vi "beam cup control - old.vi"() -> ()   [LabVIEW 2016, in "Top Level.lvlib"]
doc: "This vi is used to control the cups and apertures in the ams beamline."
uses:
  Top Level.lvlib
  sub-VIs/sub-VIs.lvlib
  controls/beamline sections.lvlib
panel:
  in  "Which Beamline":string(combo)="R45"
  out "R45 detector cup":string="OUT"
  out "R45 detector aperture":string="IN"
  out "R45 switch image cup":string="IN"
  out "R45 switch aperture":string="OUT"
  in  "R30 detector ap":bool=TRUE
  out "R30 detector aperture":string="IN"
  out "R30 Detector cup rd":string="OUT"
  out "R30 switch aperture":string="IN"
  in  "R30 Image ap":bool=TRUE
  out "R30 switch image cup":string="OUT"
  out "analyze image cup rd":string="OUT"
  out "tank exit cup  rd":string="OUT"
  out "tank entrance cup  rd":string="OUT"
  out "low energy cup":string="OUT"
  out "injector image aperture":string="IN"
  out "injector cup":string="OUT"
  in  "r45 det cup":bool
  in  "R45  det ap":bool
  in  "r45 switch image cup":bool=TRUE
  in  "R45 #1 ap":bool
  out "Terminal Voltage":dbl=8.333384070396422 format="%#_4g"
  in  "R30 det cup":bool
  in  "Switch magnet cup":bool
  in  "Analyze image cup":bool
  in  "Tank exit cup":bool
  in  "Tank Entrance cup":bool
  in  "Low end waist  cup":bool=TRUE
  in  "Low end waist ap":bool
  in  "INJ Image ap":bool
  in  "Inj Image cup":bool
  out "date/time string":string="3/16/2012  11:07 AM"
  out "Error out":errorcluster
  in  "stop":bool
  # "Faraday cup Controls"
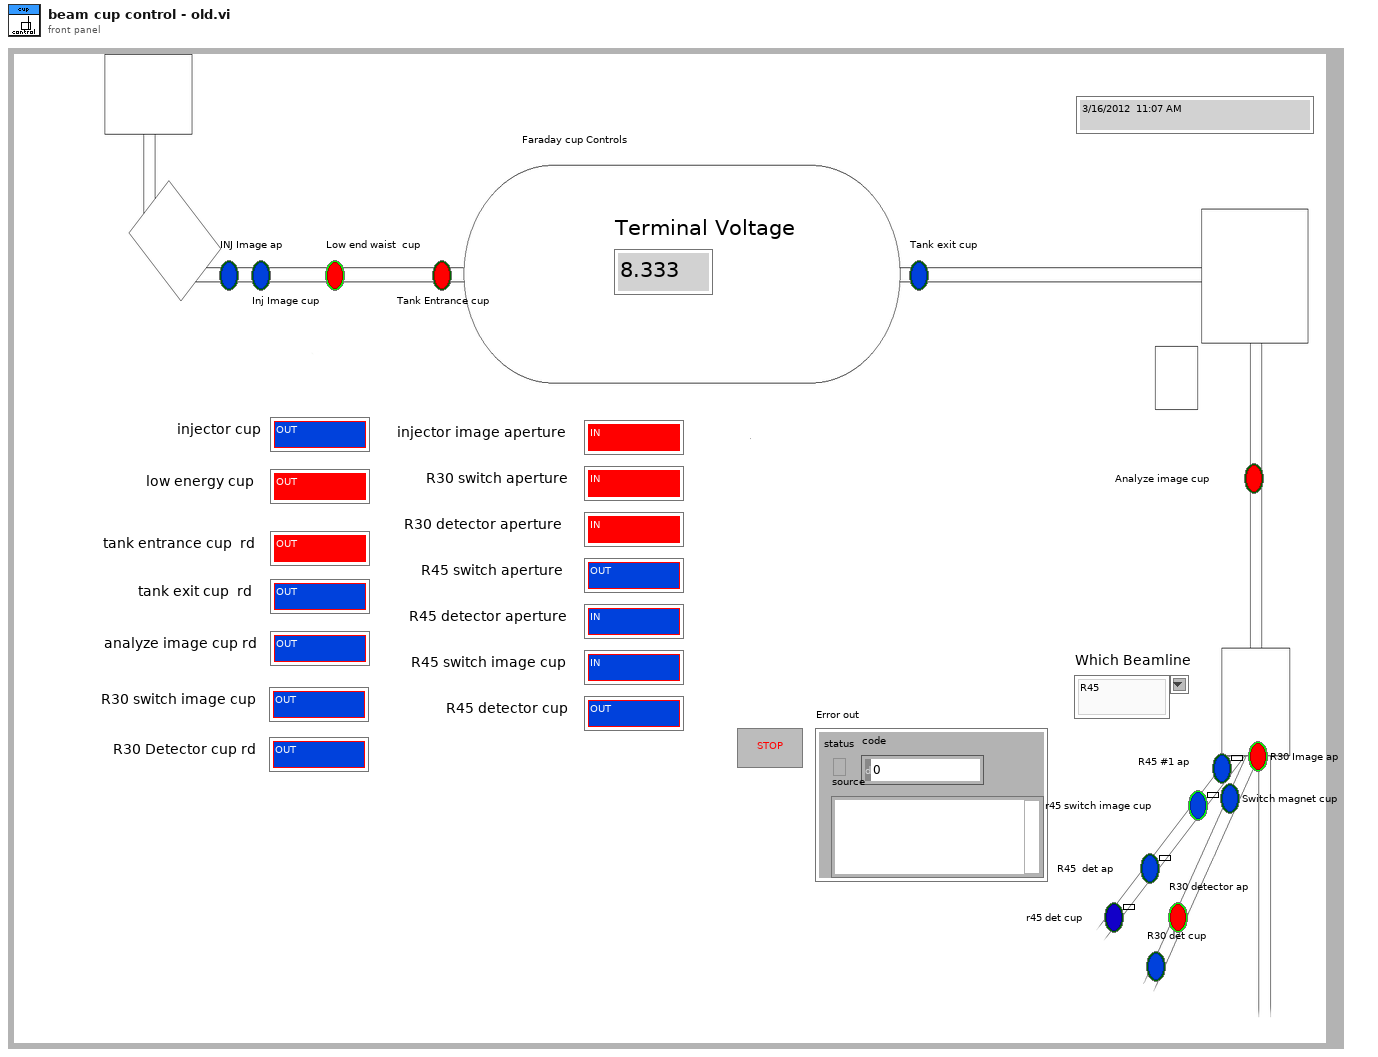
[diagram p1: front panel]
types:
  T1 = typedef "Aperture states.ctl" = enum16{"Aperture status unclear", "Aperture in", "Aperture out"}
  T2 = typedef "Faraday cup states.ctl" = enum16{"FC status unclear", "FC in", "FC out"}
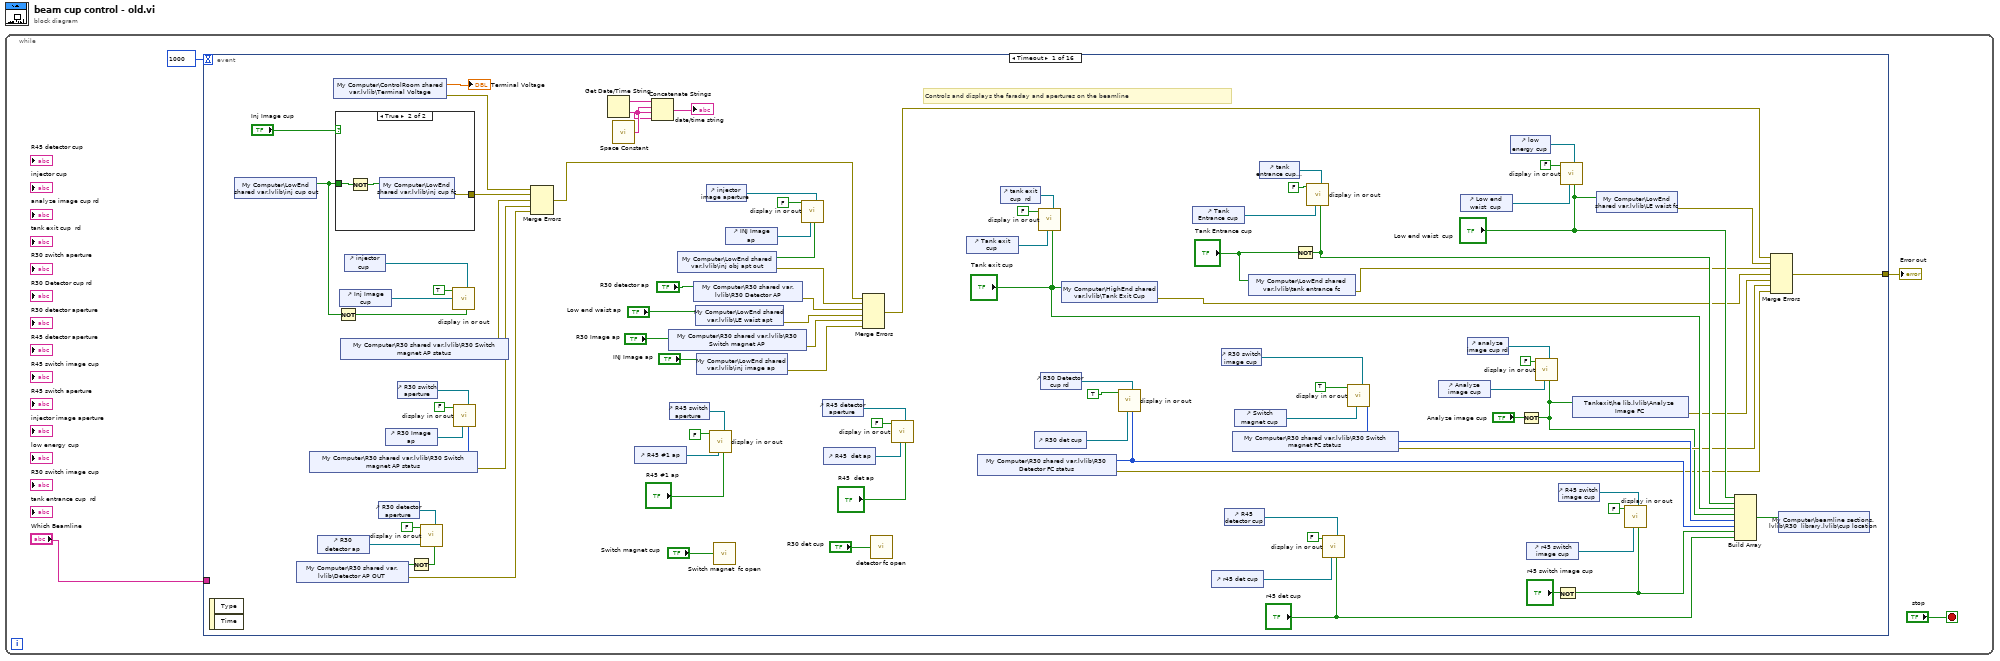
[diagram p0: block diagram]
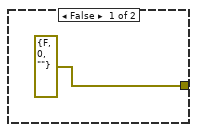
[diagram p2: hidden frame]
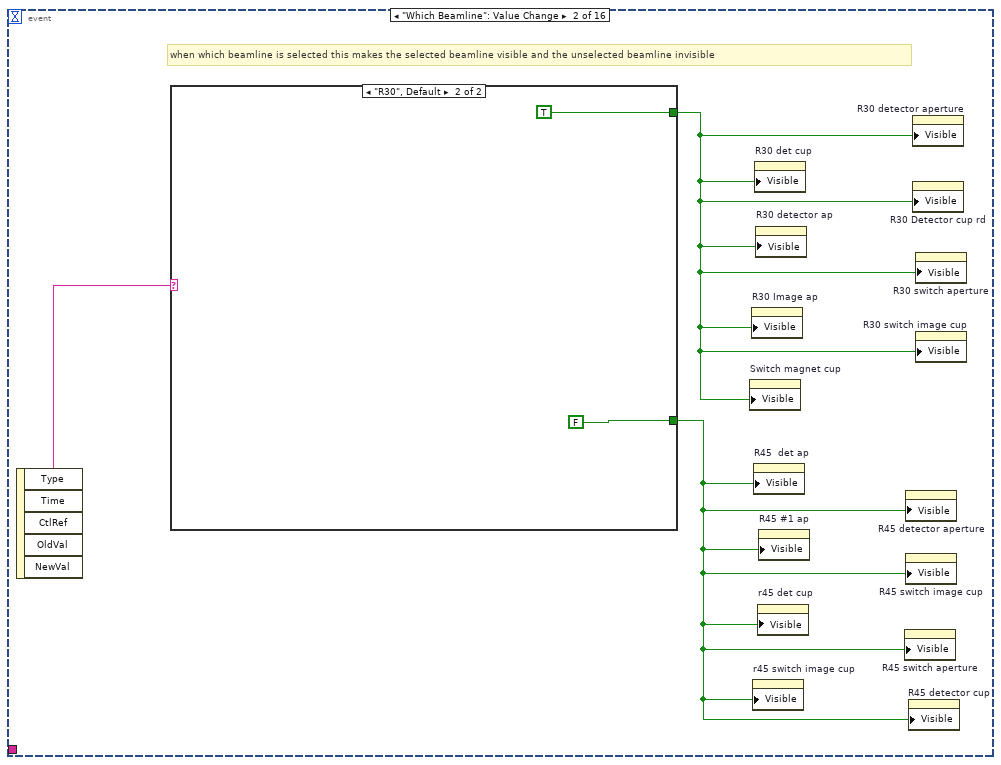
[diagram p3: hidden frame]
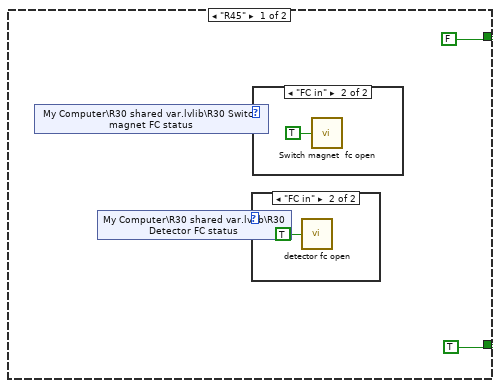
[diagram p4: hidden frame]
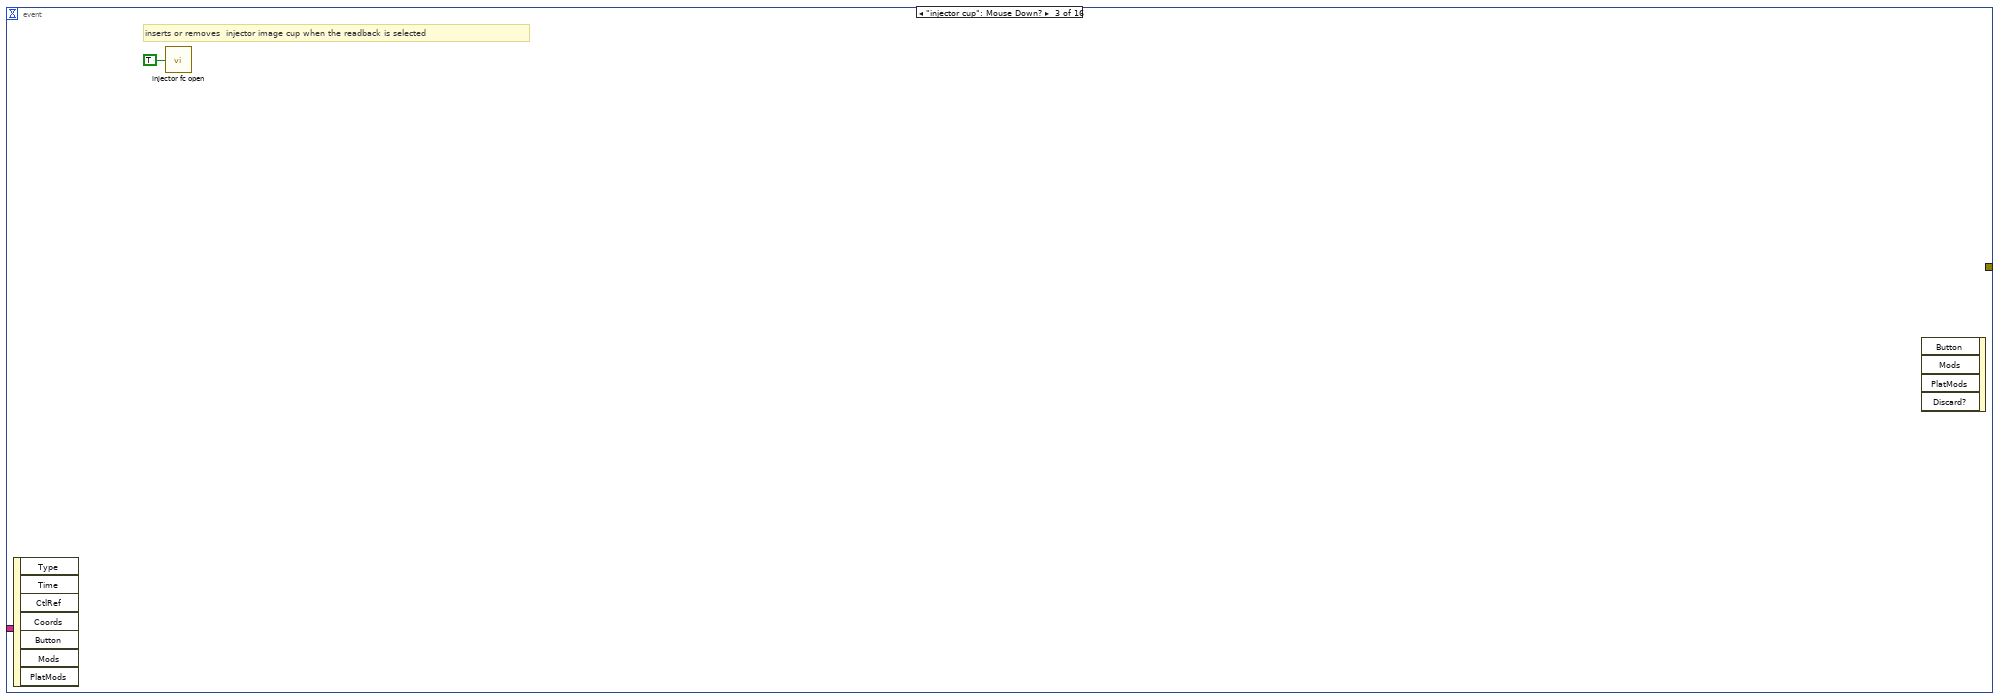
[diagram p7: hidden frame]
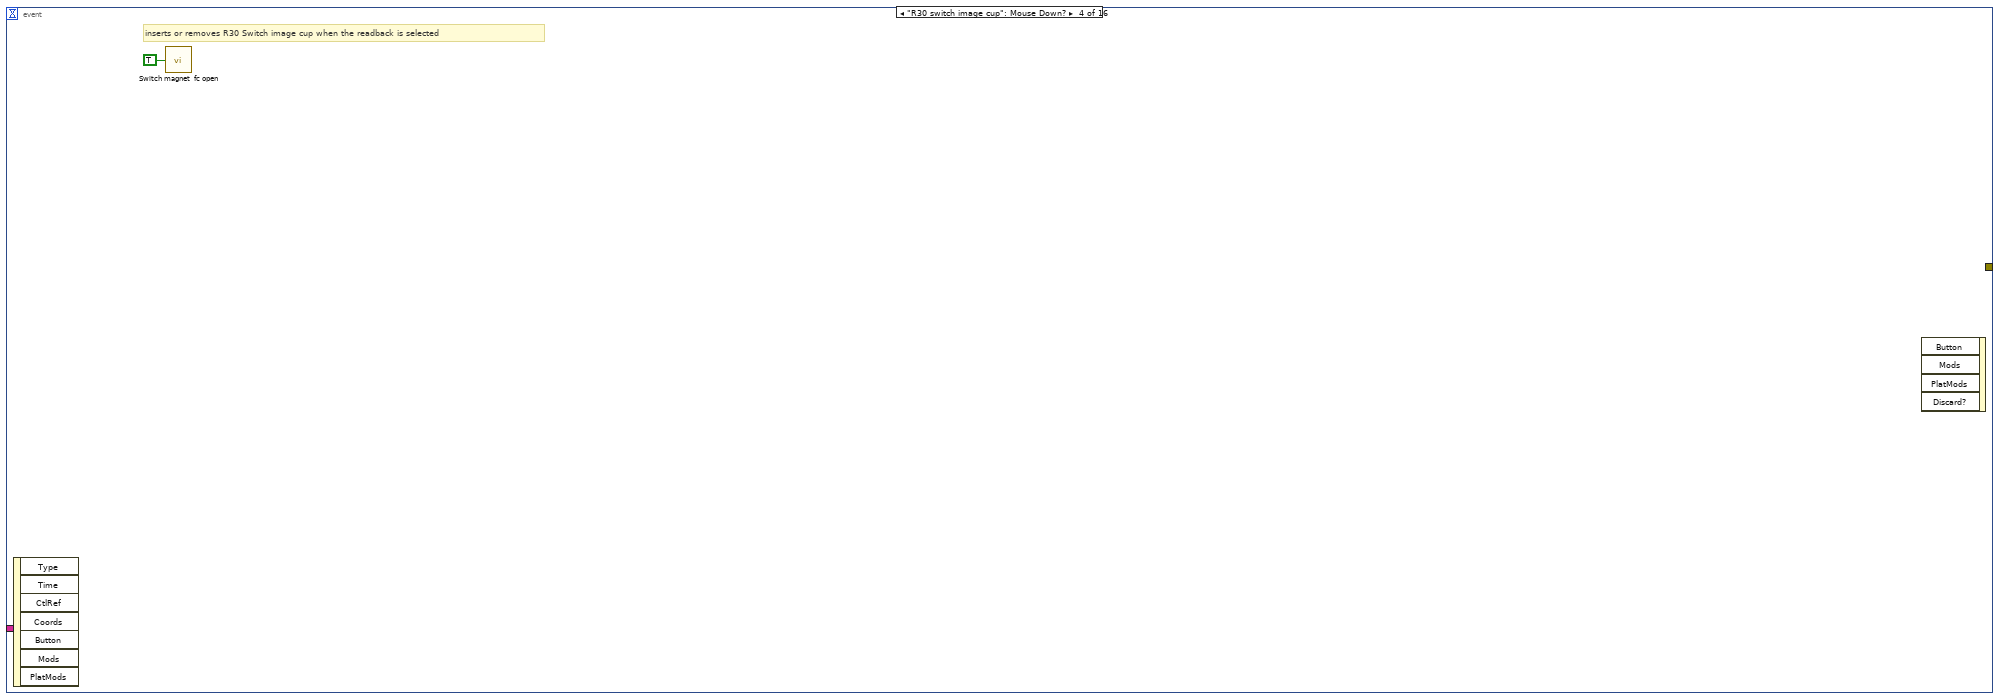
[diagram p8: hidden frame]
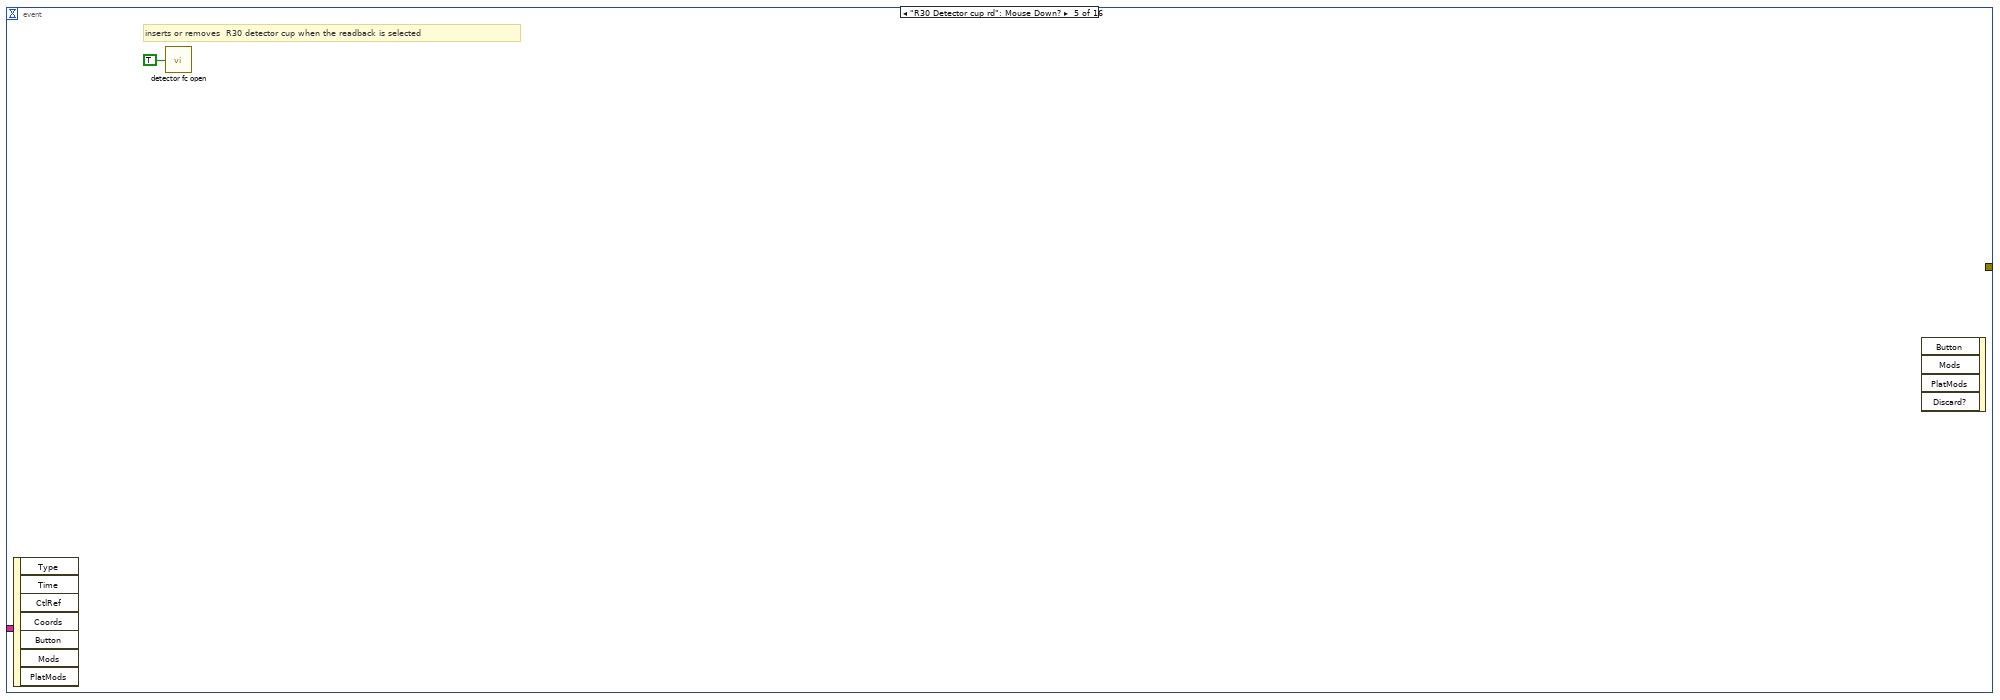
[diagram p9: hidden frame]
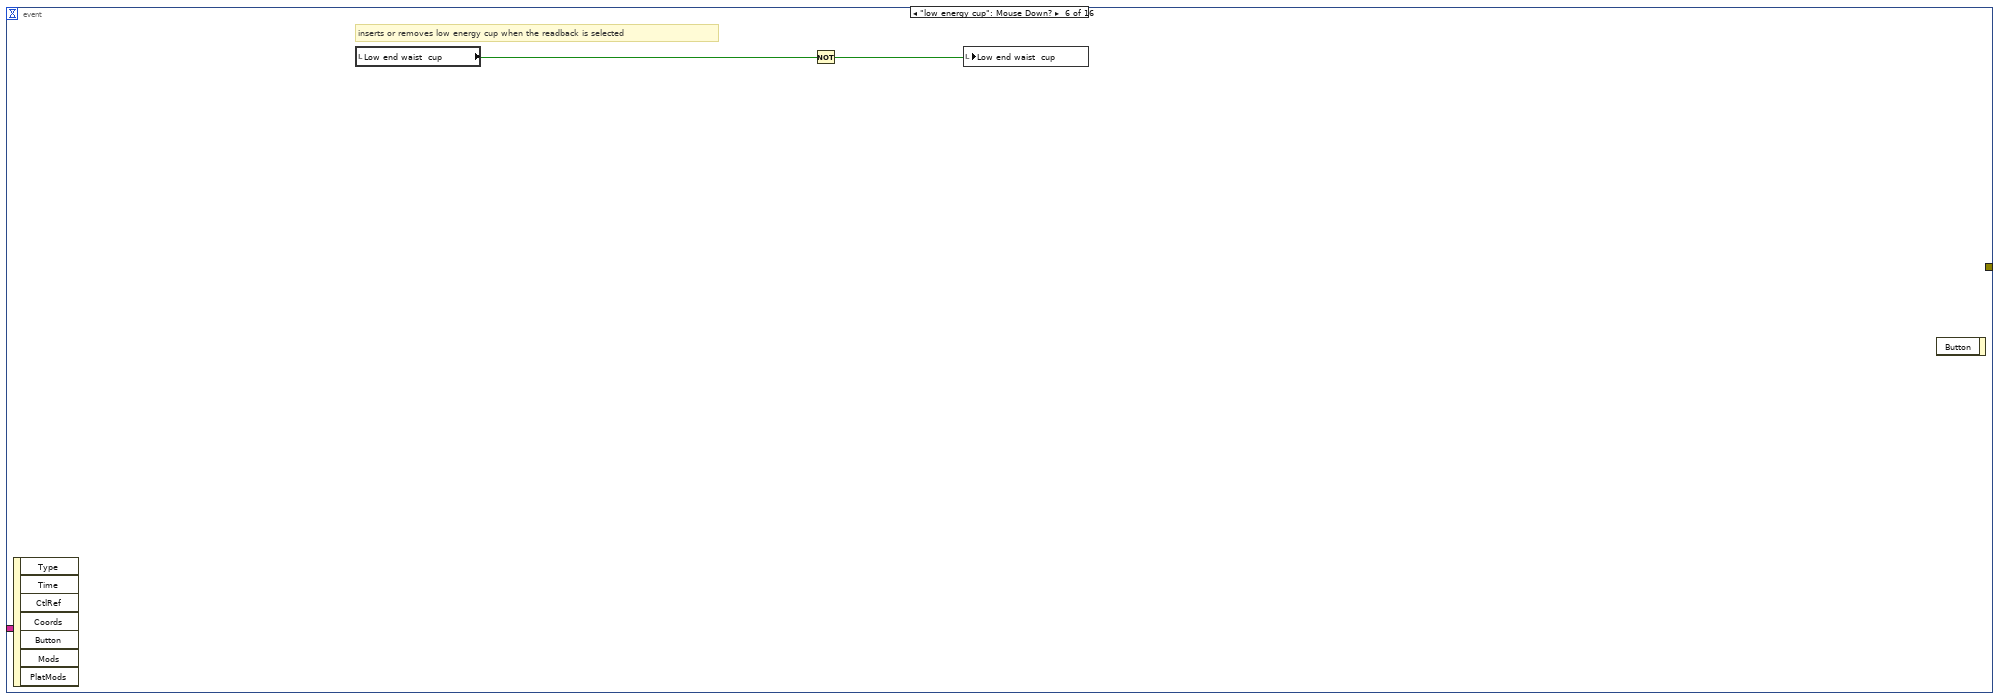
[diagram p10: hidden frame]
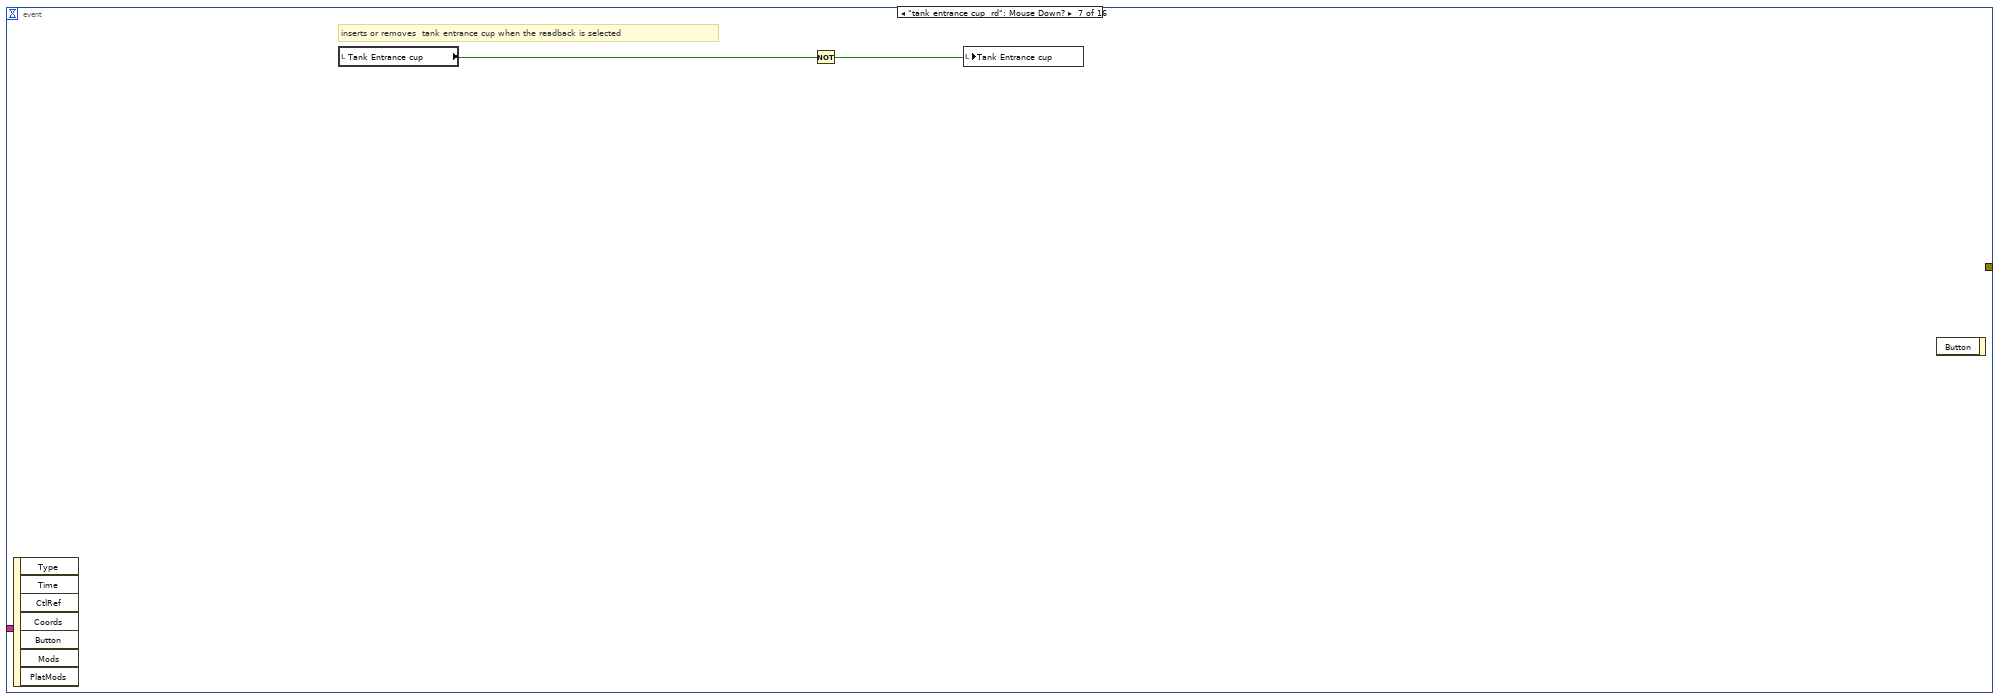
[diagram p11: hidden frame]
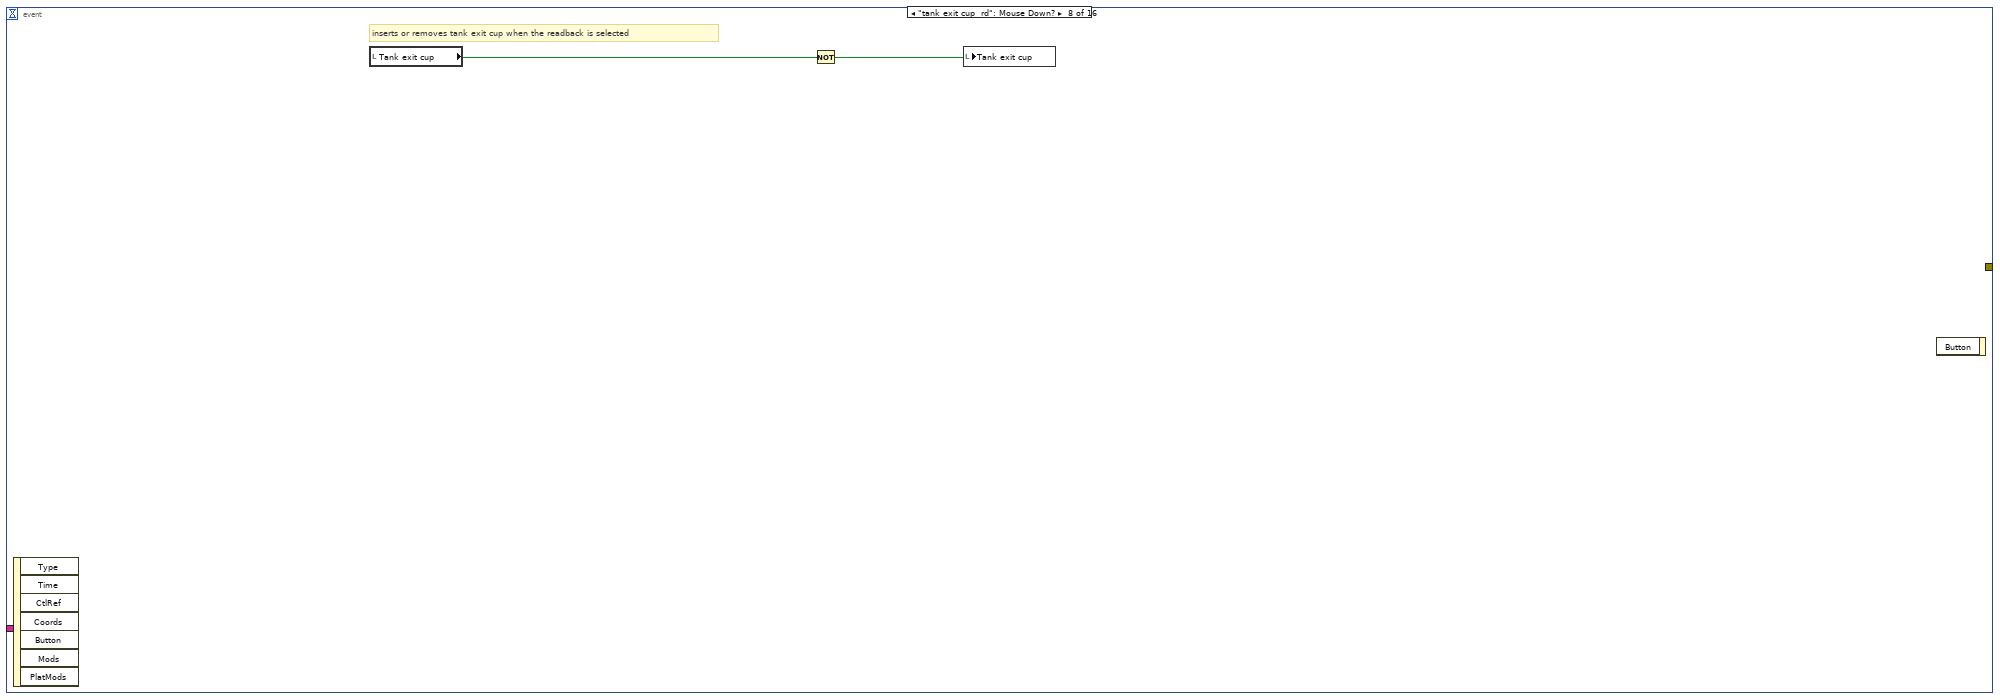
[diagram p12: hidden frame]
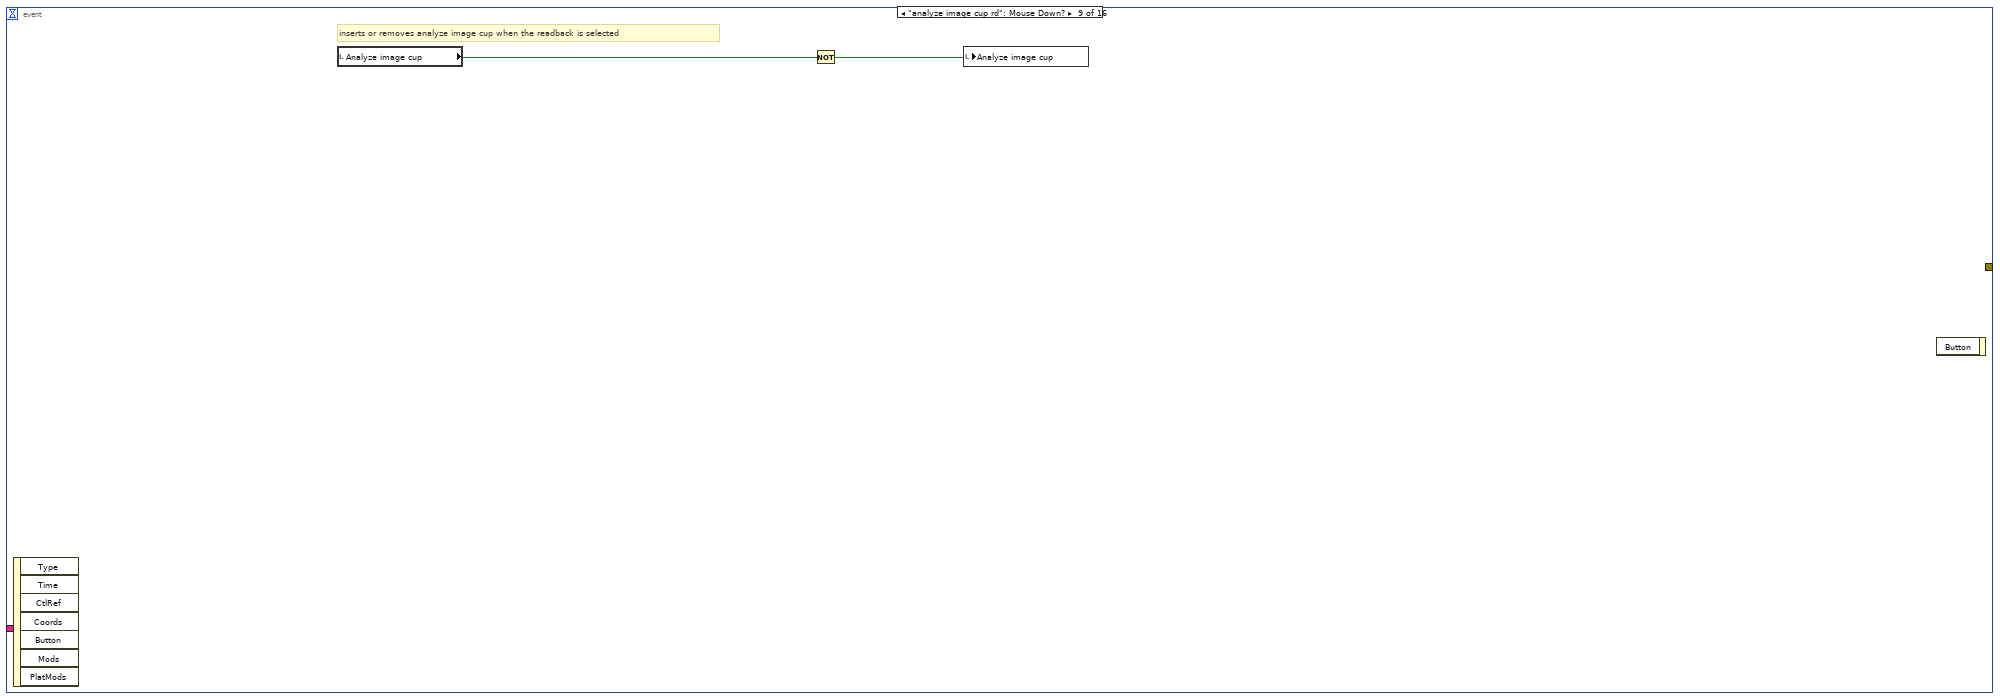
[diagram p13: hidden frame]
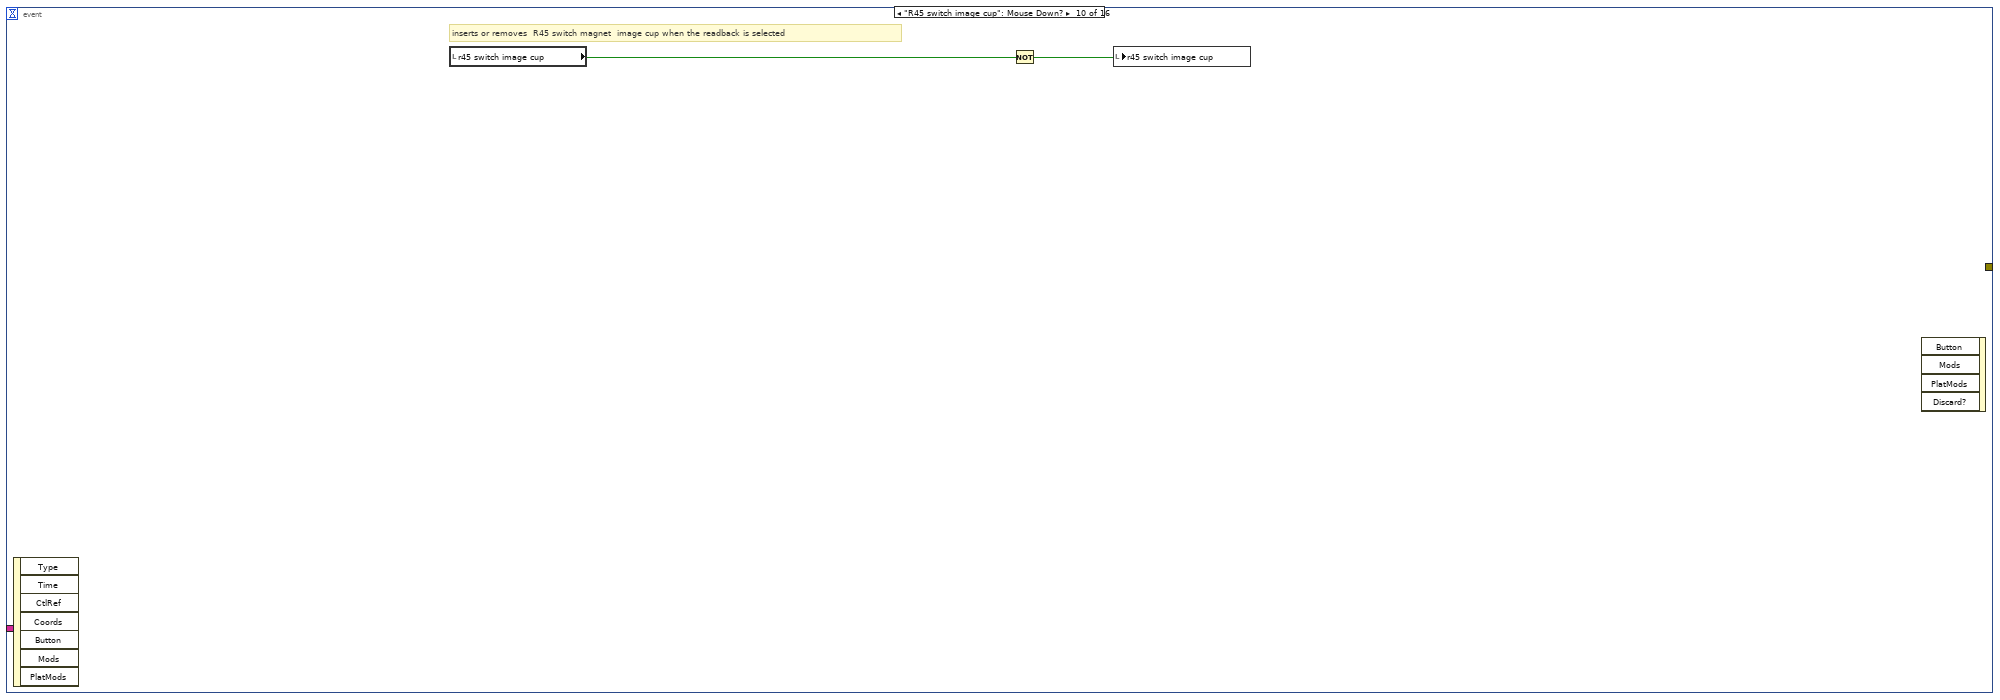
[diagram p14: hidden frame]
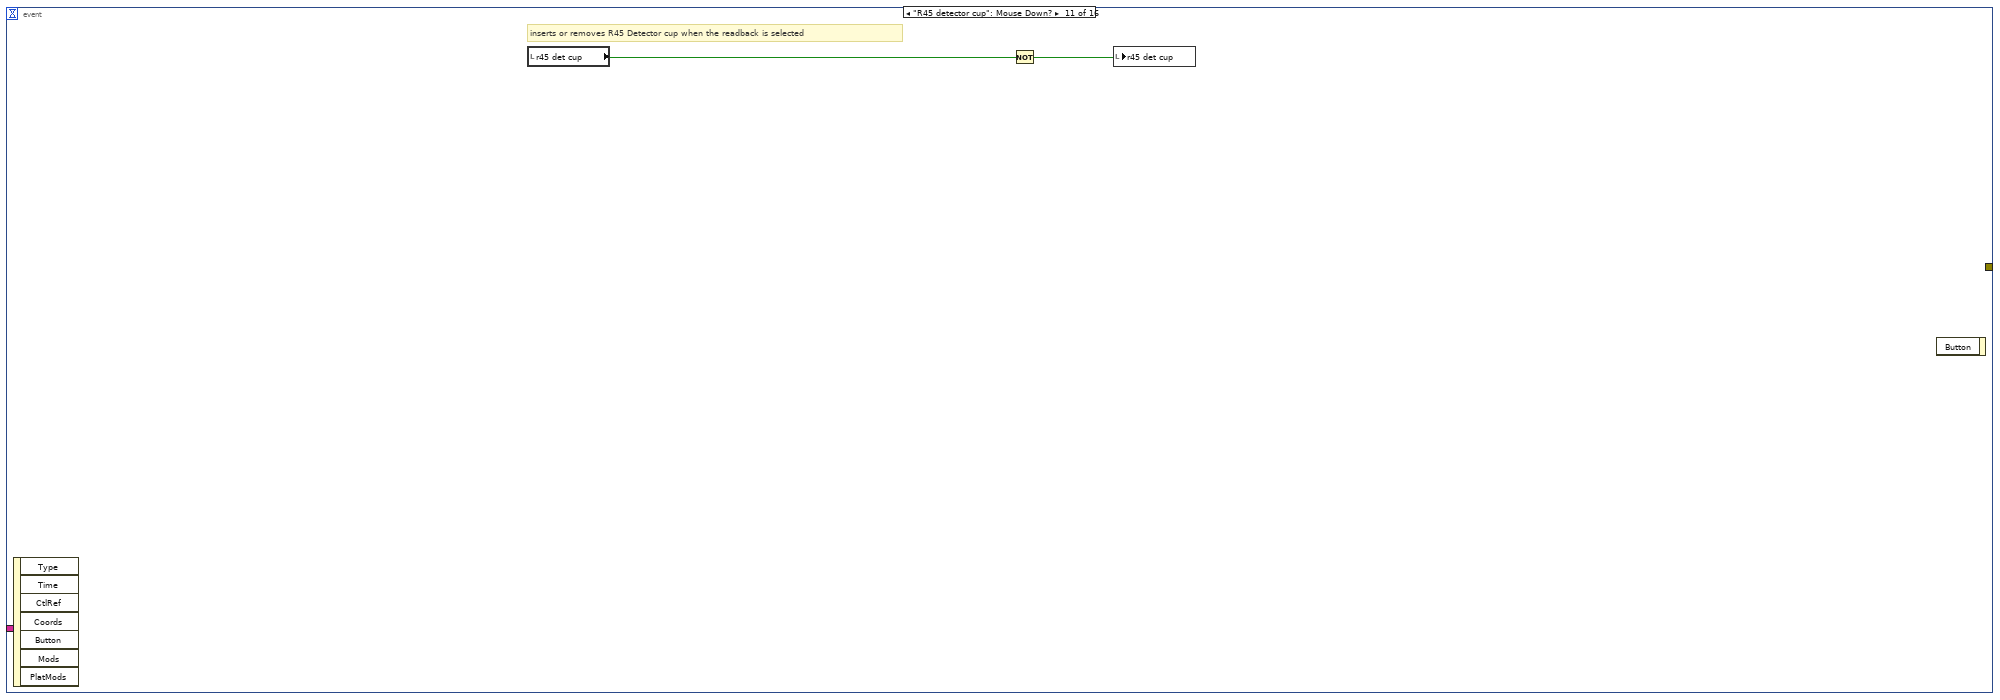
[diagram p15: hidden frame]
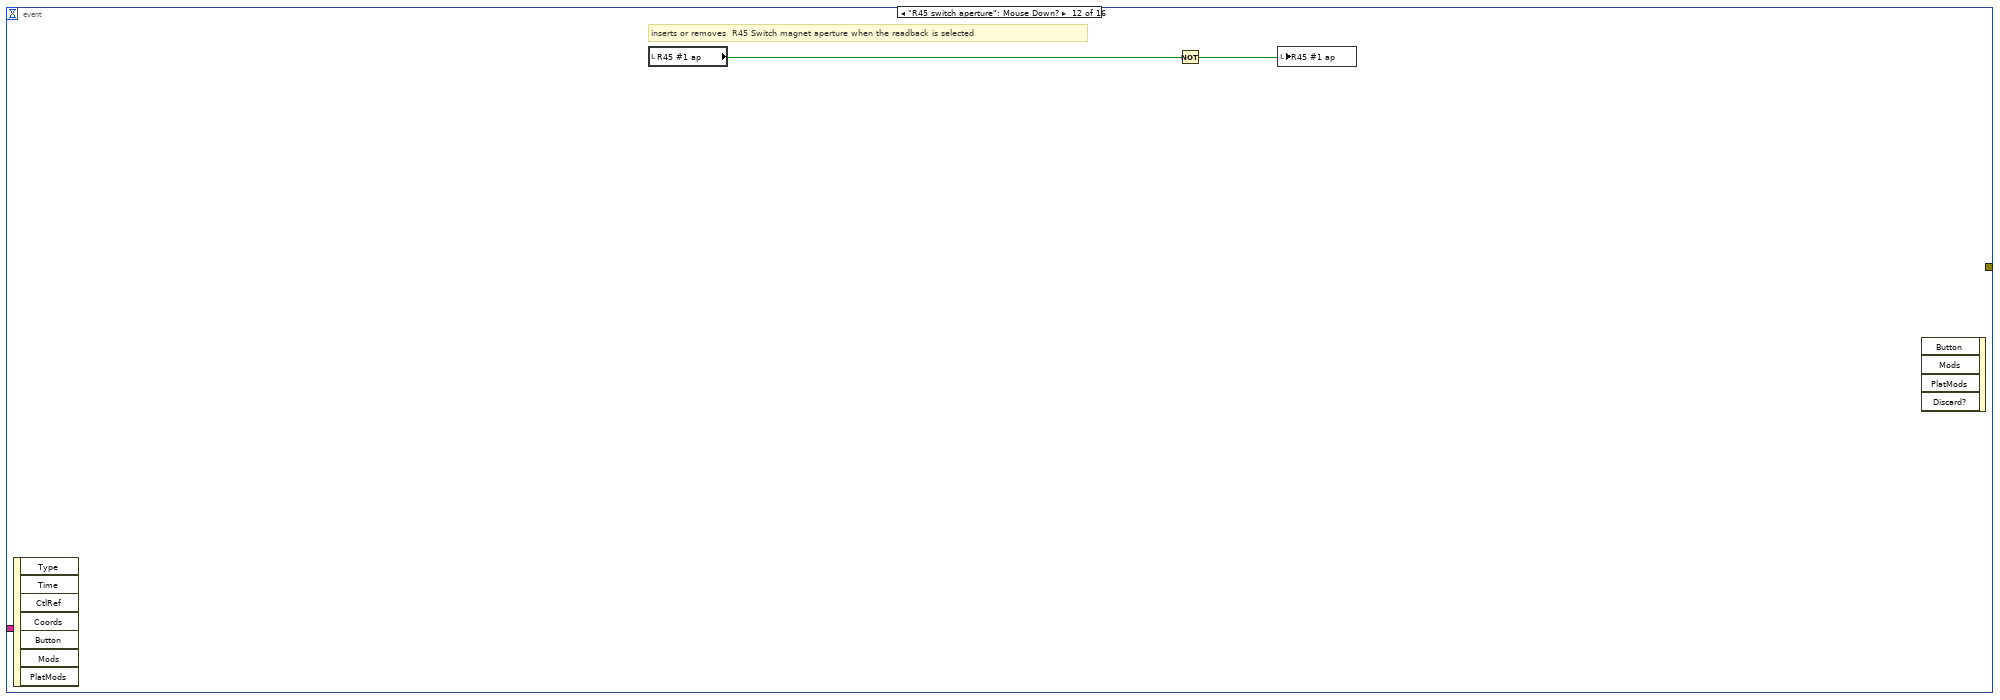
[diagram p16: hidden frame]
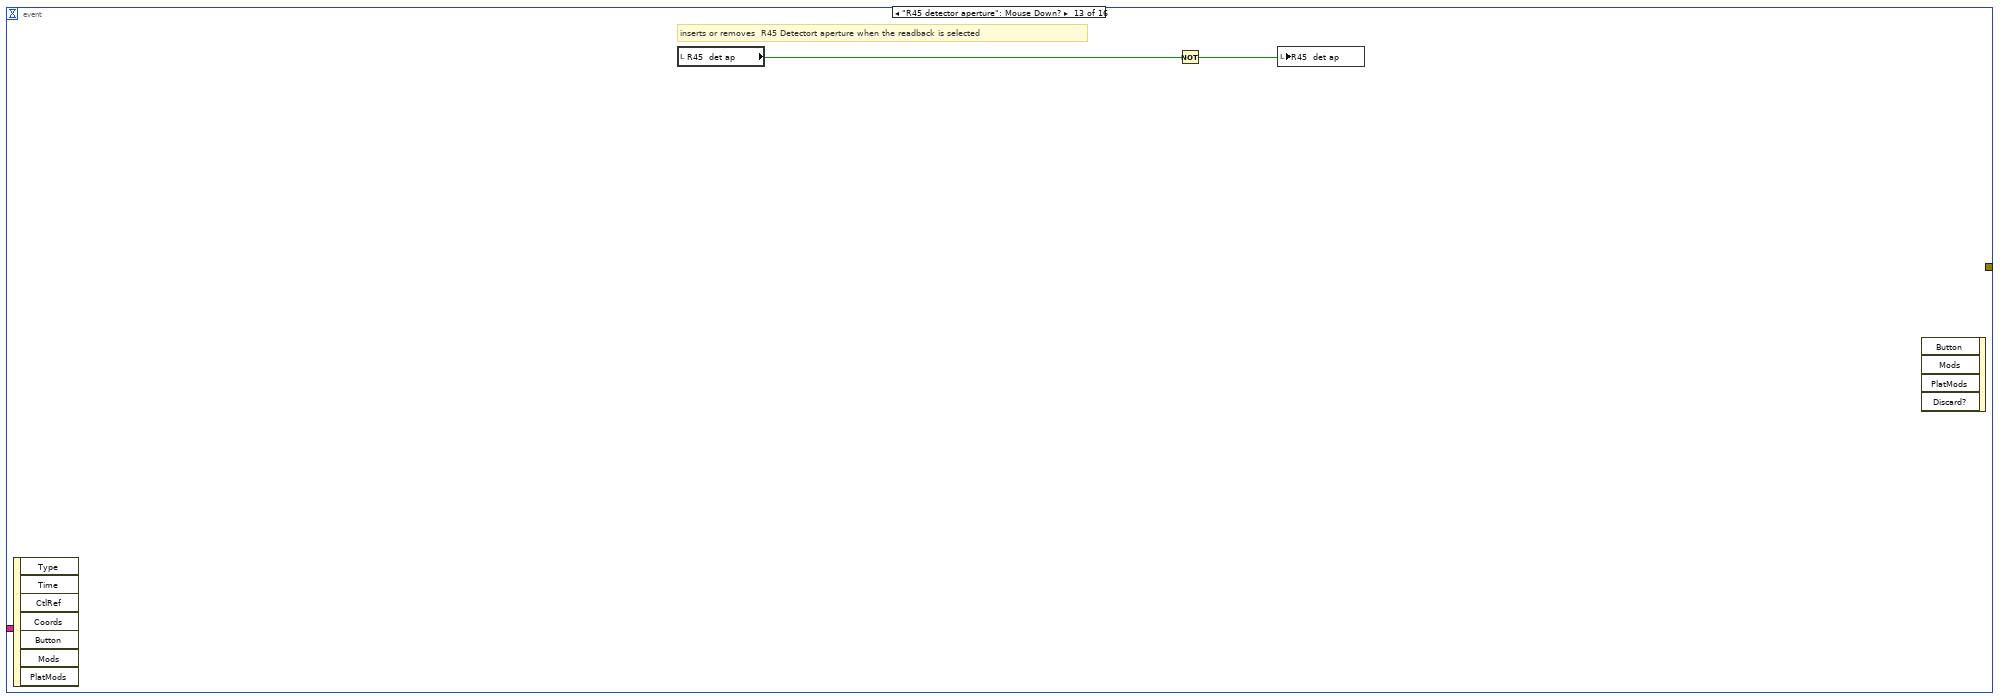
[diagram p17: hidden frame]
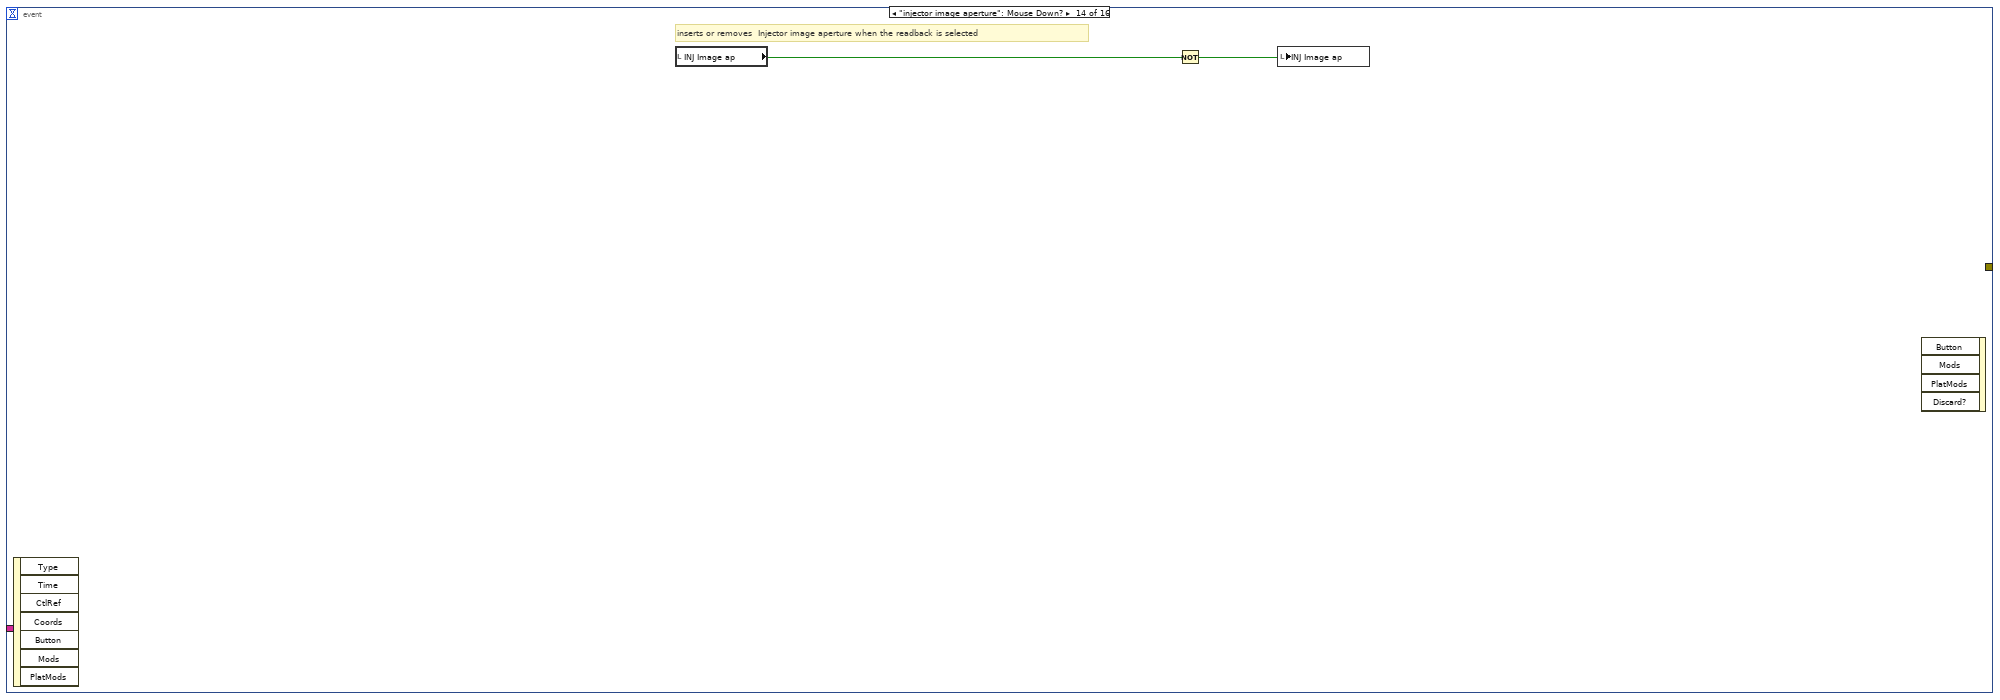
[diagram p18: hidden frame]
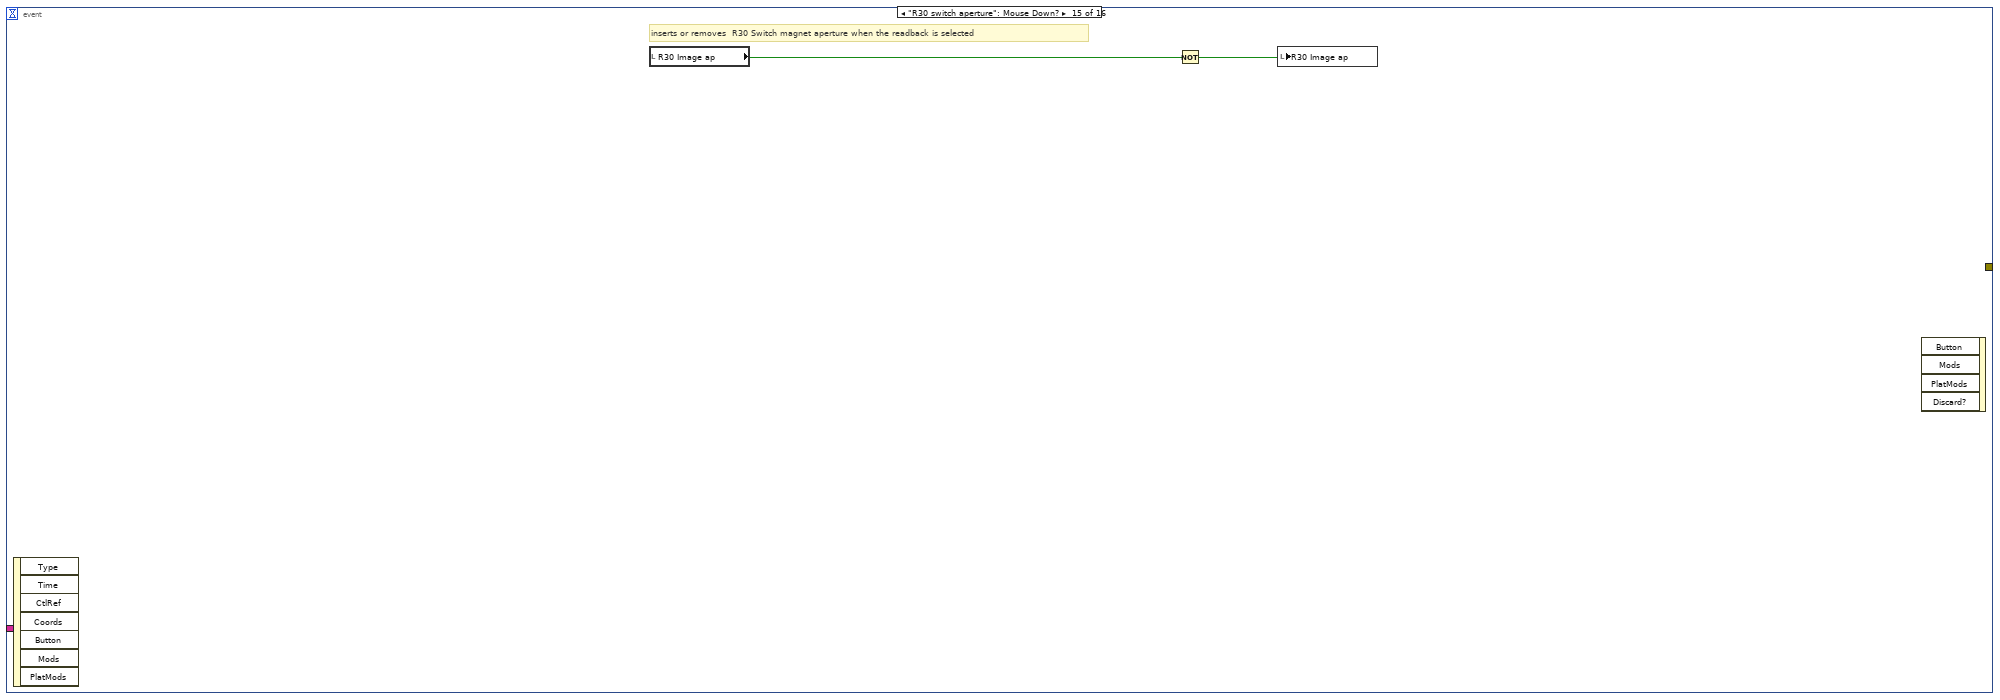
[diagram p19: hidden frame]
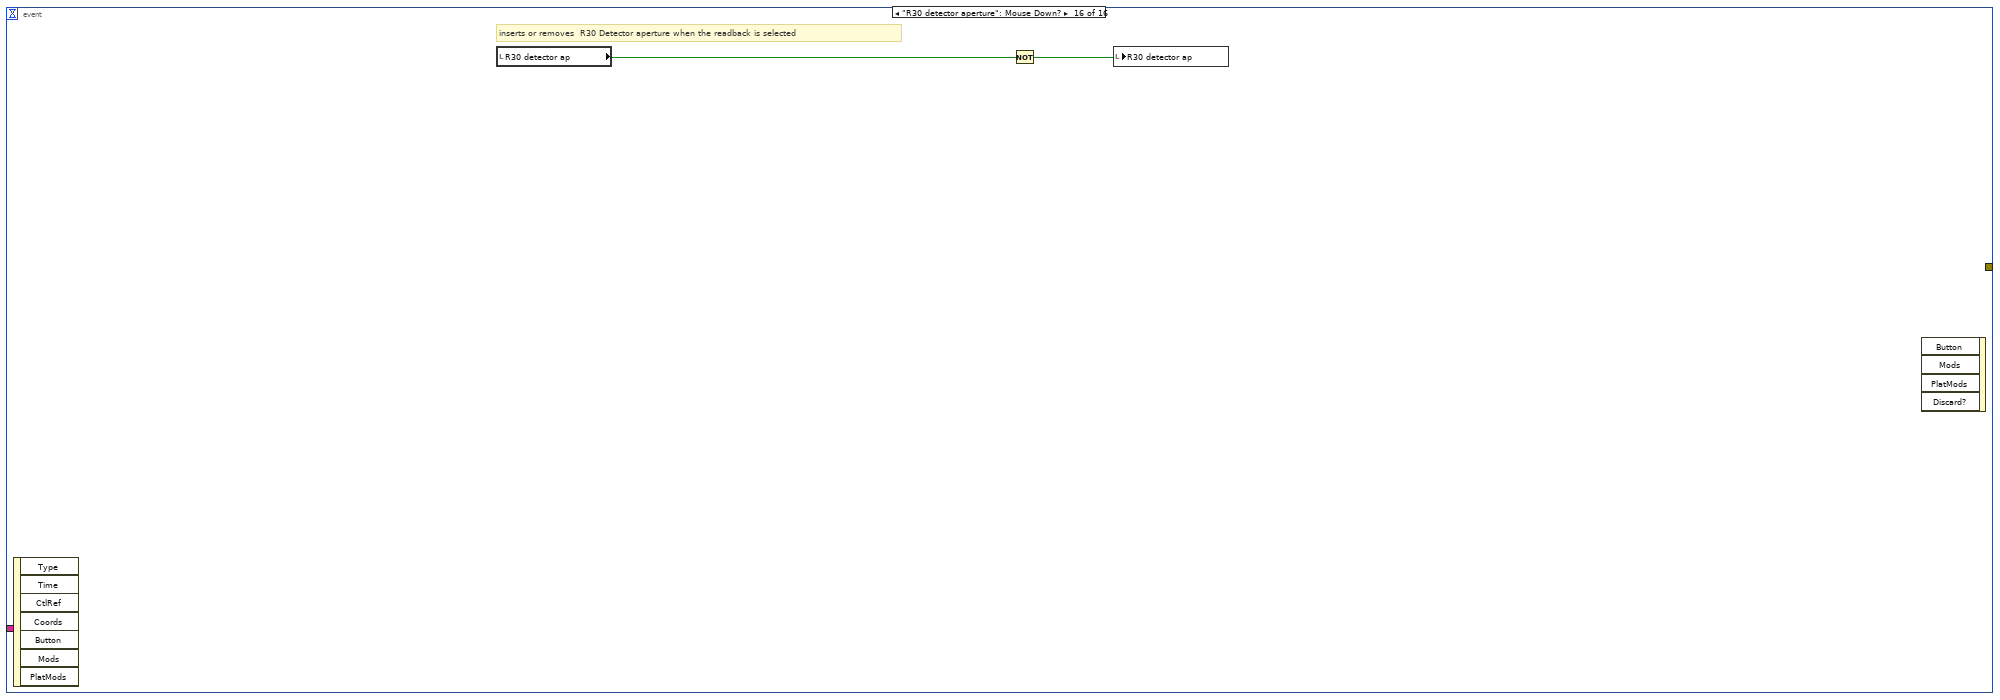
[diagram p20: hidden frame]
diagram:
  n1 = while {
    stop <- "stop" stop-if-true
    n2 = event shown="[0] Timeout" {
      selector: _ -> [_ _ _ _ _ _ _ _ _ _ _ _ _ _ _ _]
      dyn-events: _ -> [_ _ _ _ _ _ _ _ _ _ _ _ _ _ _ _]
      timeout: 1000 -> [_ _ _ _ _ _ _ _ _ _ _ _ _ _ _ _]
      tunnel: [w12 _ _ _ _ _ _ _ _ _ _ _ _ _ _ _] -> w2
      tunnel: "Which Beamline" -> [_ _ _ _ _ _ _ _ _ _ _ _ _ _ _ _]
      event Timeout {
        # "Controls and displays the faraday and apertures on the beamline"
        n3 = event-data() -> ()  [unwired: 1 in, 2 out]
        n4 = shared-variable "My Computer\\LowEnd shared var.lvlib\\inj cup out"() -> (w24:bool)  [unwired: 1 in, 1 out]
        n5 = shared-variable "My Computer\\R30 shared var.lvlib\\Detector AP OUT"() -> (w58:bool, error out=w16:errorcluster)  [unwired: 1 in]
        n6 = shared-variable "My Computer\\R30 shared var.lvlib\\R30 Switch magnet AP status"() -> (w59:T1, error out=w17:errorcluster)  [unwired: 1 in]
        n7 = control-ref of="R30 detector ap"() -> (w61:refnum<vi>)
        n8 = shared-variable "My Computer\\ControlRoom shared var.lvlib\\Terminal Voltage"() -> (→"Terminal Voltage":dbl, error out=w23:errorcluster)  [unwired: 1 in]
        n9 = case shown="True" "Inj Image cup" {
          tunnel: [errorcluster {"status"=FALSE, "code"=0, "source"=""} ("error IO") w101] -> w22
          tunnel: w24 -> [_ w100]
          frame False {
          }
          frame True {
            n10 = Not(x=w100) -> (.not. x?=w99:bool)
            n11 = shared-variable "My Computer\\LowEnd shared var.lvlib\\inj cup fc"(w99) -> (error out=w101:errorcluster)  [unwired: 1 in]
          }
        }
        n12 = Not(x=w24) -> (.not. x?=w25:bool)
        n13 = control-ref of="Inj Image cup"() -> (w92:refnum<vi>)
        n14 = shared-variable "My Computer\\R30 shared var.lvlib\\R30 Switch magnet AP status"() -> (error out=w21:errorcluster)  [unwired: 1 in, 1 out]
        n15 = control-ref of="injector cup"() -> (w93:refnum<vi>)
        n16 = control-ref of="R30 detector aperture"() -> (w60:refnum<vi>)
        n17 = control-ref of="R30 Image ap"() -> (w68:refnum<vi>)
        n18 = control-ref of="R30 switch aperture"() -> (w69:refnum<vi>)
        n19 = Not(x=w58) -> (.not. x?=w57:bool)
        n20 = call "display in or out.vi"("device in beam?"=w57, "in or out display Refnum"=w60, "device control Refnum"=w61, "use color control"=FALSE) -> ()  [unwired: 7 in, 1 out]
        n21 = call "display in or out.vi"("device in beam?"=w25, "in or out display Refnum"=w93, "device control Refnum"=w92, "use color control"=TRUE) -> ()  [unwired: 7 in, 1 out]
        n22 = call "display in or out.vi"("device in beam?"=w59, "in or out display Refnum"=w69, "device control Refnum"=w68, "use color control"=FALSE) -> ()  [unwired: 7 in, 1 out]
        n23 = Merge Errors(w23, w22, w21, w17, w16) -> (w15:errorcluster)
        n24 = Get Date/Time String() -> (date string=w97:string, time string=w94:string)  [unwired: 3 in]
        n25 = call <vilib>:"Space Constant.vi"() -> ("String"=w95:string)
        n26 = control-ref of="R45 #1 ap"() -> (w55:refnum<vi>)
        n27 = Concatenate Strings(w97, w95, w95, w94) -> (→"date/time string":string)
        n28 = shared-variable "My Computer\\R30 shared var.lvlib\\R30 Switch magnet AP"("R30 Image ap") -> (error out=w20:errorcluster)  [unwired: 1 in]
        n29 = control-ref of="R45 switch aperture"() -> (w54:refnum<vi>)
        n30 = shared-variable "My Computer\\LowEnd shared var.lvlib\\inj obj apt out"() -> (w27:bool, error out=w19:errorcluster)  [unwired: 1 in]
        n31 = shared-variable "My Computer\\R30 shared var.lvlib\\R30 Detector AP"("R30 detector ap") -> (error out=w38:errorcluster)  [unwired: 1 in]
        n32 = shared-variable "My Computer\\LowEnd shared var.lvlib\\LE waist apt"("Low end waist ap") -> (error out=w37:errorcluster)  [unwired: 1 in]
        n33 = shared-variable "My Computer\\LowEnd shared var.lvlib\\inj image ap"("INJ Image ap") -> (error out=w18:errorcluster)  [unwired: 1 in]
        n34 = control-ref of="injector image aperture"() -> (w91:refnum<vi>)
        n35 = call "display in or out.vi"("device in beam?"="R45 #1 ap", "in or out display Refnum"=w54, "device control Refnum"=w55, "use color control"=FALSE) -> ()  [unwired: 7 in, 1 out]
        n36 = call "Switch magnet  fc open.vi"("Faraday cup"="Switch magnet cup") -> ()
        n37 = control-ref of="INJ Image ap"() -> (w90:refnum<vi>)
        n38 = call "display in or out.vi"("device in beam?"=w27, "in or out display Refnum"=w91, "device control Refnum"=w90, "use color control"=FALSE) -> ()  [unwired: 7 in, 1 out]
        n39 = control-ref of="R45 detector aperture"() -> (w49:refnum<vi>)
        n40 = control-ref of="R45  det ap"() -> (w48:refnum<vi>)
        n41 = Merge Errors(w15, w19, w38, w37, w20, w18) -> (w13:errorcluster)
        n42 = call "detector fc open.vi"("Faraday cup"="R30 det cup") -> ()
        n43 = call "display in or out.vi"("device in beam?"="R45  det ap", "in or out display Refnum"=w49, "device control Refnum"=w48, "use color control"=FALSE) -> ()  [unwired: 7 in, 1 out]
        n44 = control-ref of="Tank exit cup"() -> (w79:refnum<vi>)
        n45 = shared-variable "My Computer\\R30 shared var.lvlib\\R30 Detector FC status"() -> (w63:T2, error out=w5:errorcluster)  [unwired: 1 in]
        n46 = control-ref of="tank exit cup  rd"() -> (w78:refnum<vi>)
        n47 = control-ref of="R30 det cup"() -> (w65:refnum<vi>)
        n48 = call "display in or out.vi"("device in beam?"="Tank exit cup", "in or out display Refnum"=w78, "device control Refnum"=w79, "use color control"=FALSE) -> ()  [unwired: 7 in, 1 out]
        n49 = control-ref of="R30 Detector cup rd"() -> (w66:refnum<vi>)
        n50 = shared-variable "My Computer\\HighEnd shared var.lvlib\\Tank Exit Cup"("Tank exit cup") -> (error out=w9:errorcluster)  [unwired: 1 in]
        n51 = call "display in or out.vi"("device in beam?"=w63, "in or out display Refnum"=w66, "device control Refnum"=w65, "use color control"=TRUE) -> ()  [unwired: 7 in, 1 out]
        n52 = control-ref of="Tank Entrance cup"() -> (w83:refnum<vi>)
        n53 = control-ref of="r45 det cup"() -> (w44:refnum<vi>)
        n54 = control-ref of="R30 switch image cup"() -> (w71:refnum<vi>)
        n55 = control-ref of="R45 detector cup"() -> (w43:refnum<vi>)
        n56 = shared-variable "My Computer\\R30 shared var.lvlib\\R30 Switch magnet FC status"() -> (w70:T2, error out=w7:errorcluster)  [unwired: 1 in]
        n57 = control-ref of="Switch magnet cup"() -> (w72:refnum<vi>)
        n58 = shared-variable "My Computer\\LowEnd shared var.lvlib\\tank entrance fc"("Tank Entrance cup") -> (error out=w10:errorcluster)  [unwired: 1 in]
        n59 = control-ref of="tank entrance cup  rd"() -> (w84:refnum<vi>)
        n60 = Not(x="Tank Entrance cup") -> (.not. x?=w39:bool)
        n61 = call "display in or out.vi"("device in beam?"=w39, "in or out display Refnum"=w84, "device control Refnum"=w83, "use color control"=FALSE) -> ()  [unwired: 7 in, 1 out]
        n62 = call "display in or out.vi"("device in beam?"="r45 det cup", "in or out display Refnum"=w43, "device control Refnum"=w44, "use color control"=FALSE) -> ()  [unwired: 7 in, 1 out]
        n63 = call "display in or out.vi"("device in beam?"=w70, "in or out display Refnum"=w71, "device control Refnum"=w72, "use color control"=TRUE) -> ()  [unwired: 7 in, 1 out]
        n64 = control-ref of="Analyze image cup"() -> (w75:refnum<vi>)
        n65 = control-ref of="Low end waist  cup"() -> (w86:refnum<vi>)
        n66 = control-ref of="analyze image cup rd"() -> (w76:refnum<vi>)
        n67 = control-ref of="low energy cup"() -> (w85:refnum<vi>)
        n68 = Not(x="Analyze image cup") -> (.not. x?=w6:bool)
        n69 = control-ref of="r45 switch image cup"() -> (w51:refnum<vi>)
        n70 = call "display in or out.vi"("device in beam?"=w6, "in or out display Refnum"=w76, "device control Refnum"=w75, "use color control"=FALSE) -> ()  [unwired: 7 in, 1 out]
        n71 = Not(x="r45 switch image cup") -> (.not. x?=w28:bool)
        n72 = control-ref of="R45 switch image cup"() -> (w52:refnum<vi>)
        n73 = call "display in or out.vi"("device in beam?"="Low end waist  cup", "in or out display Refnum"=w85, "device control Refnum"=w86, "use color control"=FALSE) -> ()  [unwired: 7 in, 1 out]
        n74 = shared-variable "Tankexit\\he lib.lvlib\\Analyze Image FC"(w6) -> (error out=w8:errorcluster)  [unwired: 1 in]
        n75 = shared-variable "My Computer\\LowEnd shared var.lvlib\\LE waist fc"("Low end waist  cup") -> (error out=w11:errorcluster)  [unwired: 1 in]
        n76 = call "display in or out.vi"("device in beam?"=w28, "in or out display Refnum"=w52, "device control Refnum"=w51, "use color control"=FALSE) -> ()  [unwired: 7 in, 1 out]
        n77 = Build Array("Low end waist  cup", w39, "Tank exit cup", w6, w70, w63, w28, "r45 det cup") -> (w29:bool[])
        n78 = Merge Errors(w13, w11, w10, w9, w8, w7, w5) -> (w12:errorcluster)
        n79 = shared-variable "My Computer\\beamline sections.lvlib\\R30  library.lvlib\\cup location"(w29) -> ()  [unwired: 1 in, 1 out]
      }
      event "Which Beamline": Value Change {
        # "when which beamline is selected this makes the selected beamline visible and the unselected beamline invisible"
        n80 = event-data() -> ("NewVal"=w104:string)  [unwired: 1 in, 4 out]
        n81 = case shown="\"R30\", Default" w104 {
          tunnel: [TRUE ("Visible") FALSE ("Visible")] -> w102
          tunnel: [FALSE ("Visible") TRUE ("Visible")] -> w103
          frame "R45" {
            n82 = shared-variable "My Computer\\R30 shared var.lvlib\\R30 Switch magnet FC status"() -> (w106:T2)  [unwired: 1 in, 1 out]
            n83 = shared-variable "My Computer\\R30 shared var.lvlib\\R30 Detector FC status"() -> (w105:T2)  [unwired: 1 in, 1 out]
            n84 = case shown="\"FC in\"" w105 {
              frame "FC status unclear", Default {
              }
              frame "FC in" {
                n85 = call "detector fc open.vi"("Faraday cup"=TRUE ("inj cup fc")) -> ()
              }
            }
            n86 = case shown="\"FC in\"" w106 {
              frame "FC status unclear", Default {
              }
              frame "FC in" {
                n87 = call "Switch magnet  fc open.vi"("Faraday cup"=TRUE ("inj cup fc")) -> ()
              }
            }
          }
          frame "R30", Default {
          }
        }
        n88 = property on="Switch magnet cup" class="Bool"("Visible"=w103) -> ()  [unwired: 2 in, 2 out]
        n89 = property on="R30 Image ap" class="Bool (strict)"("Visible"=w103) -> ()  [unwired: 2 in, 2 out]
        n90 = property on="r45 switch image cup" class="Bool (strict)"("Visible"=w102) -> ()  [unwired: 2 in, 2 out]
        n91 = property on="R45  det ap" class="Bool (strict)"("Visible"=w102) -> ()  [unwired: 2 in, 2 out]
        n92 = property on="R30 det cup" class="Bool"("Visible"=w103) -> ()  [unwired: 2 in, 2 out]
        n93 = property on="R30 detector ap" class="Bool (strict)"("Visible"=w103) -> ()  [unwired: 2 in, 2 out]
        n94 = property on="r45 det cup" class="Bool (strict)"("Visible"=w102) -> ()  [unwired: 2 in, 2 out]
        n95 = property on="R45 #1 ap" class="Bool (strict)"("Visible"=w102) -> ()  [unwired: 2 in, 2 out]
        n96 = property on="R45 switch aperture" class="Str"("Visible"=w102) -> ()  [unwired: 2 in, 2 out]
        n97 = property on="R45 detector aperture" class="Str"("Visible"=w102) -> ()  [unwired: 2 in, 2 out]
        n98 = property on="R45 switch image cup" class="Str"("Visible"=w102) -> ()  [unwired: 2 in, 2 out]
        n99 = property on="R45 detector cup" class="Str"("Visible"=w102) -> ()  [unwired: 2 in, 2 out]
        n100 = property on="R30 detector aperture" class="Str"("Visible"=w103) -> ()  [unwired: 2 in, 2 out]
        n101 = property on="R30 Detector cup rd" class="Str"("Visible"=w103) -> ()  [unwired: 2 in, 2 out]
        n102 = property on="R30 switch aperture" class="Str"("Visible"=w103) -> ()  [unwired: 2 in, 2 out]
        n103 = property on="R30 switch image cup" class="Str"("Visible"=w103) -> ()  [unwired: 2 in, 2 out]
      }
      event "injector cup": Mouse Down? {
        # "inserts or removes  injector image cup when the readback is selected"
        n104 = event-data() -> ()  [unwired: 1 in, 7 out]
        n105 = call "injector fc open.vi"("Faraday cup"=TRUE ("inj cup fc")) -> ()
        n106 = event-data() -> ()  [unwired: 5 in, 1 out]
      }
      event "R30 switch image cup": Mouse Down? {
        # "inserts or removes R30 Switch image cup when the readback is selected"
        n107 = event-data() -> ()  [unwired: 1 in, 7 out]
        n108 = call "Switch magnet  fc open.vi"("Faraday cup"=TRUE ("inj cup fc")) -> ()
        n109 = event-data() -> ()  [unwired: 5 in, 1 out]
      }
      event "R30 Detector cup rd": Mouse Down? {
        # "inserts or removes  R30 detector cup when the readback is selected"
        n110 = event-data() -> ()  [unwired: 1 in, 7 out]
        n111 = call "detector fc open.vi"("Faraday cup"=TRUE ("inj cup fc")) -> ()
        n112 = event-data() -> ()  [unwired: 5 in, 1 out]
      }
      event "low energy cup": Mouse Down? {
        # "inserts or removes low energy cup when the readback is selected"
        n113 = event-data() -> ()  [unwired: 1 in, 7 out]
        n114 = local read "Low end waist  cup"() -> (w117:bool)
        n115 = Not(x=w117) -> (.not. x?=w116:bool)
        n116 = local write "Low end waist  cup"(w116) -> ()
        n117 = event-data() -> ()  [unwired: 2 in, 1 out]
      }
      event "tank entrance cup  rd": Mouse Down? {
        # "inserts or removes  tank entrance cup when the readback is selected"
        n118 = event-data() -> ()  [unwired: 1 in, 7 out]
        n119 = local read "Tank Entrance cup"() -> (w119:bool)
        n120 = Not(x=w119) -> (.not. x?=w118:bool)
        n121 = local write "Tank Entrance cup"(w118) -> ()
        n122 = event-data() -> ()  [unwired: 2 in, 1 out]
      }
      event "tank exit cup  rd": Mouse Down? {
        # "inserts or removes tank exit cup when the readback is selected"
        n123 = event-data() -> ()  [unwired: 1 in, 7 out]
        n124 = local read "Tank exit cup"() -> (w121:bool)
        n125 = Not(x=w121) -> (.not. x?=w120:bool)
        n126 = local write "Tank exit cup"(w120) -> ()
        n127 = event-data() -> ()  [unwired: 2 in, 1 out]
      }
      event "analyze image cup rd": Mouse Down? {
        # "inserts or removes analyze image cup when the readback is selected"
        n128 = event-data() -> ()  [unwired: 1 in, 7 out]
        n129 = local read "Analyze image cup"() -> (w123:bool)
        n130 = Not(x=w123) -> (.not. x?=w122:bool)
        n131 = local write "Analyze image cup"(w122) -> ()
        n132 = event-data() -> ()  [unwired: 2 in, 1 out]
      }
      event "R45 switch image cup": Mouse Down? {
        # "inserts or removes  R45 switch magnet  image cup when the readback is selected"
        n133 = event-data() -> ()  [unwired: 1 in, 7 out]
        n134 = local read "r45 switch image cup"() -> (w125:bool)
        n135 = Not(x=w125) -> (.not. x?=w124:bool)
        n136 = local write "r45 switch image cup"(w124) -> ()
        n137 = event-data() -> ()  [unwired: 5 in, 1 out]
      }
      event "R45 detector cup": Mouse Down? {
        # "inserts or removes R45 Detector cup when the readback is selected"
        n138 = event-data() -> ()  [unwired: 1 in, 7 out]
        n139 = local read "r45 det cup"() -> (w127:bool)
        n140 = Not(x=w127) -> (.not. x?=w126:bool)
        n141 = local write "r45 det cup"(w126) -> ()
        n142 = event-data() -> ()  [unwired: 2 in, 1 out]
      }
      event "R45 switch aperture": Mouse Down? {
        # "inserts or removes  R45 Switch magnet aperture when the readback is selected"
        n143 = event-data() -> ()  [unwired: 1 in, 7 out]
        n144 = local read "R45 #1 ap"() -> (w129:bool)
        n145 = Not(x=w129) -> (.not. x?=w128:bool)
        n146 = local write "R45 #1 ap"(w128) -> ()
        n147 = event-data() -> ()  [unwired: 5 in, 1 out]
      }
      event "R45 detector aperture": Mouse Down? {
        # "inserts or removes  R45 Detectort aperture when the readback is selected"
        n148 = event-data() -> ()  [unwired: 1 in, 7 out]
        n149 = local read "R45  det ap"() -> (w131:bool)
        n150 = Not(x=w131) -> (.not. x?=w130:bool)
        n151 = local write "R45  det ap"(w130) -> ()
        n152 = event-data() -> ()  [unwired: 5 in, 1 out]
      }
      event "injector image aperture": Mouse Down? {
        # "inserts or removes  Injector image aperture when the readback is selected"
        n153 = event-data() -> ()  [unwired: 1 in, 7 out]
        n154 = local read "INJ Image ap"() -> (w133:bool)
        n155 = Not(x=w133) -> (.not. x?=w132:bool)
        n156 = local write "INJ Image ap"(w132) -> ()
        n157 = event-data() -> ()  [unwired: 5 in, 1 out]
      }
      event "R30 switch aperture": Mouse Down? {
        # "inserts or removes  R30 Switch magnet aperture when the readback is selected"
        n158 = event-data() -> ()  [unwired: 1 in, 7 out]
        n159 = local read "R30 Image ap"() -> (w135:bool)
        n160 = Not(x=w135) -> (.not. x?=w134:bool)
        n161 = local write "R30 Image ap"(w134) -> ()
        n162 = event-data() -> ()  [unwired: 5 in, 1 out]
      }
      event "R30 detector aperture": Mouse Down? {
        # "inserts or removes  R30 Detector aperture when the readback is selected"
        n163 = event-data() -> ()  [unwired: 1 in, 7 out]
        n164 = local read "R30 detector ap"() -> (w137:bool)
        n165 = Not(x=w137) -> (.not. x?=w136:bool)
        n166 = local write "R30 detector ap"(w136) -> ()
        n167 = event-data() -> ()  [unwired: 5 in, 1 out]
      }
    }
    "Error out" <- w2
  }
